vi "Using ParentVIRef If Input Invalid.vi"(7 "VI Ref (calling VI)":refnum<vi>) -> (2 "Using Parent Ref(Need to Destroy)":bool, 3 "VI Ref":refnum<vi>)   [LabVIEW 2017]
doc: "This utility will fit (resize and center) a VI (defined by the \"VI Ref\" input) about the largest decoration in that VI. It will add a border defined by border spacing in units of pixels. If there are no decorations found in the VI it is a no-op and will not produce an error. Unfortunately, this VI can not find locked decorations (yet)."
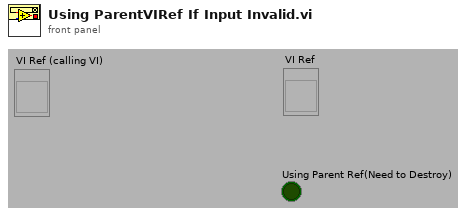
[diagram p1: front panel]
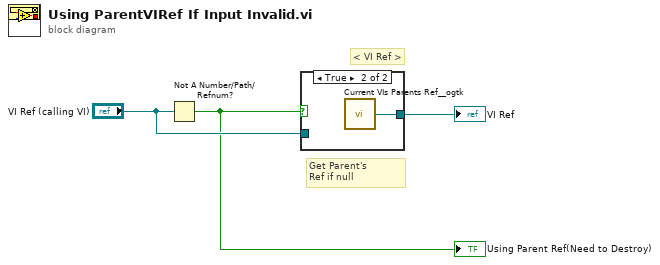
[diagram p0: block diagram]
diagram:
  # "Get Parent's\nRef if null"
  # "< VI Ref >"
  n1 = Not A Number/Path/Refnum?(number/path/refnum="VI Ref (calling VI)") -> (NaN/Path/Refnum?=w1:bool)
  "Using Parent Ref(Need to Destroy)" <- w1
  n2 = case shown="True" w1 {
    tunnel: [w4 w5] -> w2
    tunnel: "VI Ref (calling VI)" -> [w4 _]
    frame False {
    }
    frame True {
      n3 = call <userlib>:"Current VIs Parents Ref__ogtk.vi"() -> ("Calling VI's Reference"=w5:refnum<vi>)  [unwired: 2 in]
    }
  }
  "VI Ref" <- w2
